vi "TrapezoidalMotionProfile.vi"(5 "MaxAccel":dbl=75.0, 7 "MaxVelocity":dbl=100.0, 8 "dt":u32=20, 9 "FinalVelocity":dbl, 10 "InitialVelocity":dbl, 11 "Distance":dbl=200.0) -> (0 "dt":u32=20, 1 "Accel":dbl[](array[numeric])=[0.0, 1.5, 3.0, 4.5, 6.0, 7.5, 9.0, 10.500000000000002, 12.0, 13.5, 15.0, 16.5, 18.0, 19.5, 21.000000000000004, 22.5, 24.0, 25.500000000000004, 27.0, 28.5, 30.0, 31.5, 33.0, 34.5, 36.0, 37.5, 39.0, 40.5, 42.00000000000001, 43.5, 45.0, 46.5, 48.0, 49.5, 51.00000000000001, 52.50000000000001, 54.0, 55.5, 57.0, 58.5, 60.0, 61.50000000000001, 63.0, 64.5, 66.0, 67.5, 69.0, 70.5, 72.0, 73.5, 75.0, 76.5, 78.0, 79.5, 81.0, 82.5, 84.00000000000001, 85.50000000000001, 87.0, 88.5, 90.0, 91.5, 93.0, 94.5, 96.0, 97.5, 99.0, 100.0, 100.0, 100.0, 100.0, 100.0, 100.0, 100.0, 100.0, 100.0, 100.0, 100.0, 100.0, 100.0, 100.0, 100.0, 100.0, 100.0, 100.0, 100.0, 100.0, 100.0, 100.0, 100.0, 100.0, 100.0, 100.0, 100.0, 100.0, 100.0, 100.0, 100.0, 100.0, 100.0, 100.0, 98.5, 97.0, 95.5, 94.0, 92.5, 91.0, 89.49999999999999, 87.99999999999999, 86.49999999999999, 84.99999999999999, 83.49999999999999, 81.99999999999999, 80.49999999999999, 78.99999999999999, 77.49999999999997, 76.00000000000001, 74.50000000000001, 73.00000000000001, 71.5, 70.0, 68.5, 67.0, 65.5, 64.0, 62.5, 61.0, 59.5, 57.99999999999999, 56.49999999999999, 54.99999999999999, 53.49999999999999, 51.99999999999999, 50.499999999999986, 48.999999999999986, 47.499999999999986, 45.999999999999986, 44.499999999999986, 42.999999999999986, 41.49999999999998, 39.99999999999998, 38.500000000000014, 37.000000000000014, 35.500000000000014, 34.000000000000014, 32.5, 31.0, 29.5, 28.0, 26.5, 25.0, 23.5, 22.0, 20.5, 19.0, 17.5, 15.999999999999986, 14.499999999999986, 12.999999999999986, 11.499999999999986, 9.999999999999986, 8.499999999999986, 6.999999999999986, 5.499999999999986, 3.999999999999986, 2.499999999999986, 0.9999999999999716, -0.4999999999999858], 2 "Vel":dbl[](array[numeric])=[0.0, 1.5, 3.0, 4.5, 6.0, 7.5, 9.0, 10.500000000000002, 12.0, 13.5, 15.0, 16.5, 18.0, 19.5, 21.000000000000004, 22.5, 24.0, 25.500000000000004, 27.0, 28.5, 30.0, 31.5, 33.0, 34.5, 36.0, 37.5, 39.0, 40.5, 42.00000000000001, 43.5, 45.0, 46.5, 48.0, 49.5, 51.00000000000001, 52.50000000000001, 54.0, 55.5, 57.0, 58.5, 60.0, 61.50000000000001, 63.0, 64.5, 66.0, 67.5, 69.0, 70.5, 72.0, 73.5, 75.0, 76.5, 78.0, 79.5, 81.0, 82.5, 84.00000000000001, 85.50000000000001, 87.0, 88.5, 90.0, 91.5, 93.0, 94.5, 96.0, 97.5, 99.0, 100.0, 100.0, 100.0, 100.0, 100.0, 100.0, 100.0, 100.0, 100.0, 100.0, 100.0, 100.0, 100.0, 100.0, 100.0, 100.0, 100.0, 100.0, 100.0, 100.0, 100.0, 100.0, 100.0, 100.0, 100.0, 100.0, 100.0, 100.0, 100.0, 100.0, 100.0, 100.0, 100.0, 100.0, 98.5, 97.0, 95.5, 94.0, 92.5, 91.0, 89.49999999999999, 87.99999999999999, 86.49999999999999, 84.99999999999999, 83.49999999999999, 81.99999999999999, 80.49999999999999, 78.99999999999999, 77.49999999999997, 76.00000000000001, 74.50000000000001, 73.00000000000001, 71.5, 70.0, 68.5, 67.0, 65.5, 64.0, 62.5, 61.0, 59.5, 57.99999999999999, 56.49999999999999, 54.99999999999999, 53.49999999999999, 51.99999999999999, 50.499999999999986, 48.999999999999986, 47.499999999999986, 45.999999999999986, 44.499999999999986, 42.999999999999986, 41.49999999999998, 39.99999999999998, 38.500000000000014, 37.000000000000014, 35.500000000000014, 34.000000000000014, 32.5, 31.0, 29.5, 28.0, 26.5, 25.0, 23.5, 22.0, 20.5, 19.0, 17.5, 15.999999999999986, 14.499999999999986, 12.999999999999986, 11.499999999999986, 9.999999999999986, 8.499999999999986, 6.999999999999986, 5.499999999999986, 3.999999999999986, 2.499999999999986, 0.9999999999999716, -0.4999999999999858], 3 "Pos":dbl[](array[numeric])=[0.0, 0.015000000000000001, 0.060000000000000005, 0.135, 0.24000000000000002, 0.37500000000000006, 0.54, 0.7350000000000001, 0.9600000000000001, 1.2149999999999999, 1.5000000000000002, 1.815, 2.16, 2.535, 2.9400000000000004, 3.375, 3.8400000000000003, 4.335000000000001, 4.859999999999999, 5.415, 6.000000000000001, 6.614999999999999, 7.26, 7.9350000000000005, 8.64, 9.375, 10.14, 10.935, 11.760000000000002, 12.614999999999998, 13.5, 14.415000000000001, 15.360000000000001, 16.335, 17.340000000000003, 18.375000000000004, 19.439999999999998, 20.535, 21.66, 22.815, 24.000000000000004, 25.215000000000003, 26.459999999999997, 27.734999999999996, 29.04, 30.375000000000004, 31.740000000000002, 33.135000000000005, 34.56, 36.015, 37.5, 39.015, 40.56, 42.135000000000005, 43.74, 45.37500000000001, 47.040000000000006, 48.735000000000014, 50.459999999999994, 52.214999999999996, 54.0, 55.815, 57.660000000000004, 59.535000000000004, 61.440000000000005, 63.37500000000001, 65.34, 67.33333333333334, 69.33333333333334, 71.33333333333334, 73.33333333333334, 75.33333333333333, 77.33333333333333, 79.33333333333333, 81.33333333333333, 83.33333333333333, 85.33333333333333, 87.33333333333334, 89.33333333333334, 91.33333333333334, 93.33333333333334, 95.33333333333334, 97.33333333333334, 99.33333333333334, 101.33333333333333, 103.33333333333333, 105.33333333333333, 107.33333333333333, 109.33333333333333, 111.33333333333334, 113.33333333333334, 115.33333333333334, 117.33333333333334, 119.33333333333334, 121.33333333333334, 123.33333333333334, 125.33333333333331, 127.33333333333333, 129.33333333333331, 131.33333333333331, 133.33333333333331, 135.31833333333338, 137.27333333333337, 139.19833333333338, 141.09333333333336, 142.95833333333337, 144.79333333333338, 146.59833333333336, 148.37333333333336, 150.11833333333337, 151.83333333333337, 153.51833333333337, 155.17333333333337, 156.79833333333337, 158.39333333333337, 159.95833333333337, 161.49333333333334, 162.99833333333333, 164.47333333333336, 165.91833333333335, 167.33333333333334, 168.71833333333336, 170.07333333333335, 171.39833333333334, 172.69333333333336, 173.95833333333334, 175.19333333333336, 176.39833333333337, 177.57333333333335, 178.71833333333336, 179.83333333333334, 180.91833333333335, 181.97333333333336, 182.99833333333336, 183.99333333333337, 184.95833333333334, 185.89333333333335, 186.79833333333335, 187.67333333333335, 188.51833333333335, 189.33333333333334, 190.11833333333334, 190.87333333333333, 191.59833333333333, 192.29333333333335, 192.95833333333334, 193.59333333333333, 194.19833333333335, 194.77333333333334, 195.31833333333333, 195.83333333333334, 196.31833333333333, 196.77333333333334, 197.19833333333335, 197.59333333333333, 197.95833333333334, 198.29333333333335, 198.59833333333333, 198.87333333333333, 199.11833333333334, 199.33333333333334, 199.51833333333335, 199.67333333333335, 199.79833333333335, 199.89333333333335, 199.95833333333334, 199.99333333333334, 199.99833333333333])   [LabVIEW 2016]
panel:
  out "Graph":dbl[][](graph)=[[0.0, 0.015000000000000001, 0.060000000000000005, 0.135, 0.24000000000000002, 0.37500000000000006, 0.54, 0.7350000000000001, 0.9600000000000001, 1.2149999999999999, 1.5000000000000002, 1.815, 2.16, 2.535, 2.9400000000000004, 3.375, 3.8400000000000003, 4.335000000000001, 4.859999999999999, 5.415, 6.000000000000001, 6.614999999999999, 7.26, 7.9350000000000005, 8.64, 9.375, 10.14, 10.935, 11.760000000000002, 12.614999999999998, 13.5, 14.415000000000001, 15.360000000000001, 16.335, 17.340000000000003, 18.375000000000004, 19.439999999999998, 20.535, 21.66, 22.815, 24.000000000000004, 25.215000000000003, 26.459999999999997, 27.734999999999996, 29.04, 30.375000000000004, 31.740000000000002, 33.135000000000005, 34.56, 36.015, 37.5, 39.015, 40.56, 42.135000000000005, 43.74, 45.37500000000001, 47.040000000000006, 48.735000000000014, 50.459999999999994, 52.214999999999996, 54.0, 55.815, 57.660000000000004, 59.535000000000004, 61.440000000000005, 63.37500000000001, 65.34, 67.33333333333334, 69.33333333333334, 71.33333333333334, 73.33333333333334, 75.33333333333333, 77.33333333333333, 79.33333333333333, 81.33333333333333, 83.33333333333333, 85.33333333333333, 87.33333333333334, 89.33333333333334, 91.33333333333334, 93.33333333333334, 95.33333333333334, 97.33333333333334, 99.33333333333334, 101.33333333333333, 103.33333333333333, 105.33333333333333, 107.33333333333333, 109.33333333333333, 111.33333333333334, 113.33333333333334, 115.33333333333334, 117.33333333333334, 119.33333333333334, 121.33333333333334, 123.33333333333334, 125.33333333333331, 127.33333333333333, 129.33333333333331, 131.33333333333331, 133.33333333333331, 135.31833333333338, 137.27333333333337, 139.19833333333338, 141.09333333333336, 142.95833333333337, 144.79333333333338, 146.59833333333336, 148.37333333333336, 150.11833333333337, 151.83333333333337, 153.51833333333337, 155.17333333333337, 156.79833333333337, 158.39333333333337, 159.95833333333337, 161.49333333333334, 162.99833333333333, 164.47333333333336, 165.91833333333335, 167.33333333333334, 168.71833333333336, 170.07333333333335, 171.39833333333334, 172.69333333333336, 173.95833333333334, 175.19333333333336, 176.39833333333337, 177.57333333333335, 178.71833333333336, 179.83333333333334, 180.91833333333335, 181.97333333333336, 182.99833333333336, 183.99333333333337, 184.95833333333334, 185.89333333333335, 186.79833333333335, 187.67333333333335, 188.51833333333335, 189.33333333333334, 190.11833333333334, 190.87333333333333, 191.59833333333333, 192.29333333333335, 192.95833333333334, 193.59333333333333, 194.19833333333335, 194.77333333333334, 195.31833333333333, 195.83333333333334, 196.31833333333333, 196.77333333333334, 197.19833333333335, 197.59333333333333, 197.95833333333334, 198.29333333333335, 198.59833333333333, 198.87333333333333, 199.11833333333334, 199.33333333333334, 199.51833333333335, 199.67333333333335, 199.79833333333335, 199.89333333333335, 199.95833333333334, 199.99333333333334, 199.99833333333333], [0.0, 1.5, 3.0, 4.5, 6.0, 7.5, 9.0, 10.500000000000002, 12.0, 13.5, 15.0, 16.5, 18.0, 19.5, 21.000000000000004, 22.5, 24.0, 25.500000000000004, 27.0, 28.5, 30.0, 31.5, 33.0, 34.5, 36.0, 37.5, 39.0, 40.5, 42.00000000000001, 43.5, 45.0, 46.5, 48.0, 49.5, 51.00000000000001, 52.50000000000001, 54.0, 55.5, 57.0, 58.5, 60.0, 61.50000000000001, 63.0, 64.5, 66.0, 67.5, 69.0, 70.5, 72.0, 73.5, 75.0, 76.5, 78.0, 79.5, 81.0, 82.5, 84.00000000000001, 85.50000000000001, 87.0, 88.5, 90.0, 91.5, 93.0, 94.5, 96.0, 97.5, 99.0, 100.0, 100.0, 100.0, 100.0, 100.0, 100.0, 100.0, 100.0, 100.0, 100.0, 100.0, 100.0, 100.0, 100.0, 100.0, 100.0, 100.0, 100.0, 100.0, 100.0, 100.0, 100.0, 100.0, 100.0, 100.0, 100.0, 100.0, 100.0, 100.0, 100.0, 100.0, 100.0, 100.0, 100.0, 98.5, 97.0, 95.5, 94.0, 92.5, 91.0, 89.49999999999999, 87.99999999999999, 86.49999999999999, 84.99999999999999, 83.49999999999999, 81.99999999999999, 80.49999999999999, 78.99999999999999, 77.49999999999997, 76.00000000000001, 74.50000000000001, 73.00000000000001, 71.5, 70.0, 68.5, 67.0, 65.5, 64.0, 62.5, 61.0, 59.5, 57.99999999999999, 56.49999999999999, 54.99999999999999, 53.49999999999999, 51.99999999999999, 50.499999999999986, 48.999999999999986, 47.499999999999986, 45.999999999999986, 44.499999999999986, 42.999999999999986, 41.49999999999998, 39.99999999999998, 38.500000000000014, 37.000000000000014, 35.500000000000014, 34.000000000000014, 32.5, 31.0, 29.5, 28.0, 26.5, 25.0, 23.5, 22.0, 20.5, 19.0, 17.5, 15.999999999999986, 14.499999999999986, 12.999999999999986, 11.499999999999986, 9.999999999999986, 8.499999999999986, 6.999999999999986, 5.499999999999986, 3.999999999999986, 2.499999999999986, 0.9999999999999716, -0.4999999999999858]]
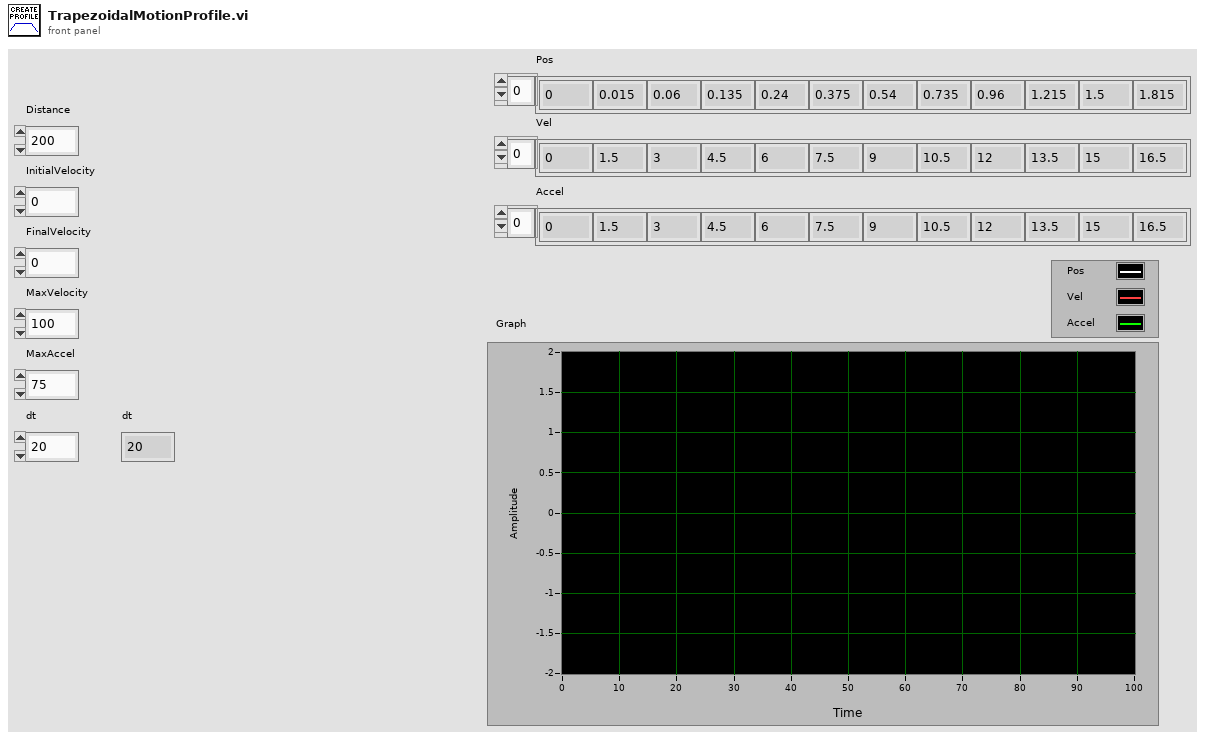
[diagram p1: front panel]
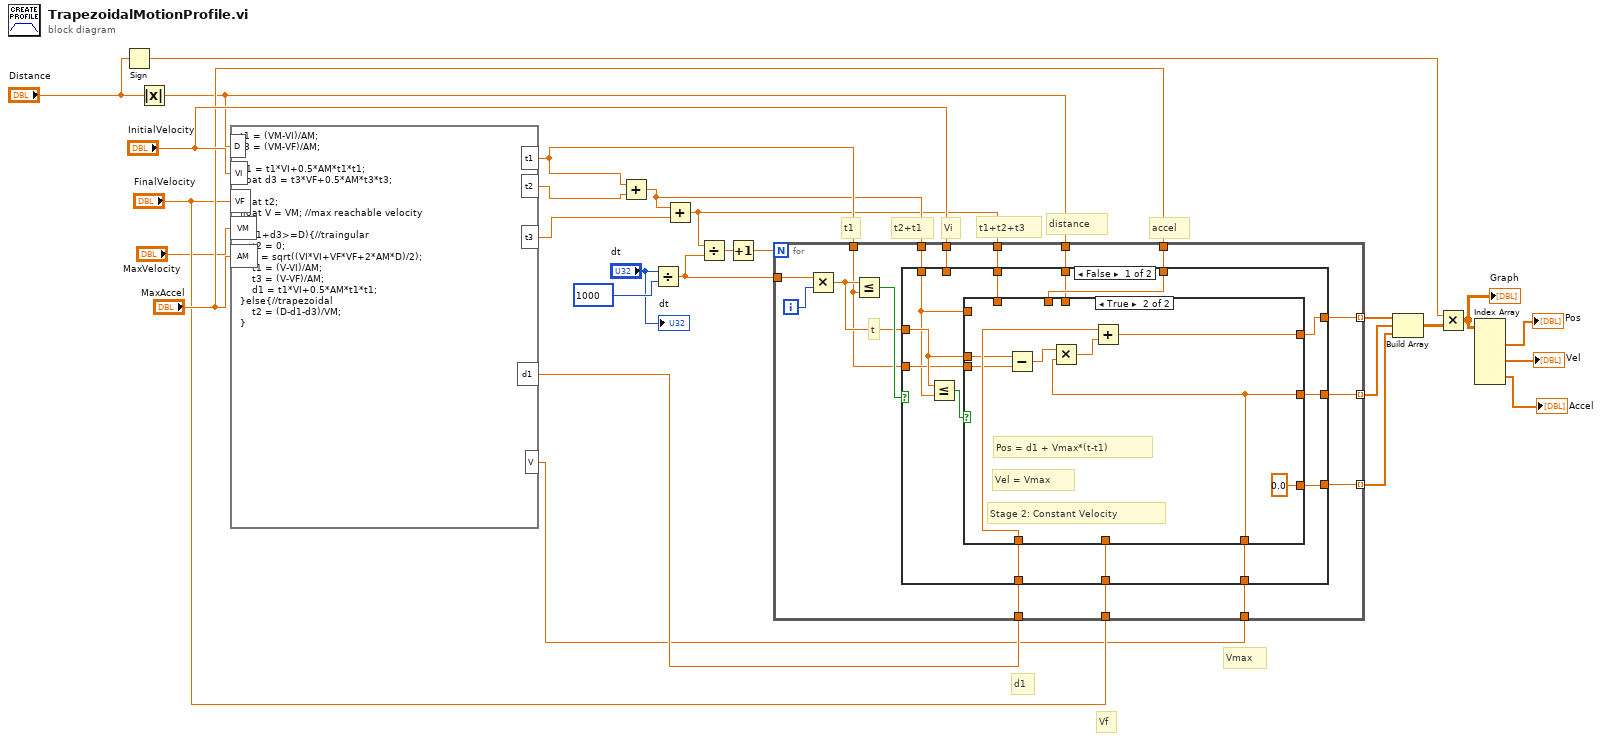
[diagram p0: block diagram]
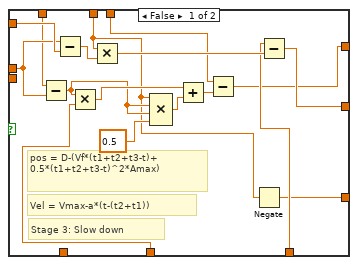
[diagram p2: hidden frame]
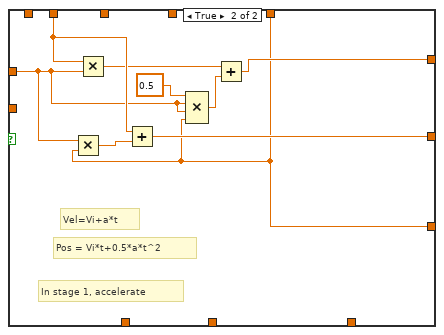
[diagram p3: hidden frame]
diagram:
  # "distance"
  # "Vf"
  # "t1+t2+t3"
  # "d1"
  # "Vmax"
  # "t1"
  # "t2+t1"
  # "Vi"
  # "accel"
  n1 = Sign(1:"Distance") -> (0:w5:dbl)
  n2 = Absolute Value(x="Distance") -> (abs(x)=w8:dbl)
  n3 = formula code="t1 = (VM-VI)/AM;\nt3 = (VM-VF)/AM;\n\nd1 = t1*VI+0.5*AM*t1*t1;\nfloat d3 = t3*VF+0.5*AM*t3*t3;\n\nfloat t2;\nfloat V = VM; //max reachable velocity\n\nif(d1+d3>=D){//traingular\n    t2 = 0;\n    V = sqrt((VI*VI+VF*VF+2*AM*D)/2);\n    t1 = (V-VI)/AM;\n    t3 = (V-VF)/AM;\n    d1 = t1*VI+0.5*AM*t1*t1;\n}else{//trapezoidal\n    t2 = (D-d1-d3)/VM;\n}"("VI"="InitialVelocity", "VF"="FinalVelocity", "D"=w8, "VM"="MaxVelocity", "AM"="MaxAccel") -> ("t1"=w21:dbl, "t3"=w26:dbl, "d1"=w17:dbl, "t2"=w27:dbl, "V"=w10:dbl)
  n4 = Add(x=w21, y=w27) -> (x+y=w18:dbl)
  n5 = Divide(x="dt", y=u32 1000) -> (x/y=w22:dbl)
  n6 = Add(x=w18, y=w26) -> (x+y=w14:dbl)
  n7 = Divide(x=w14, y=w22) -> (x/y=w24:dbl)
  n8 = Increment(x=w24) -> (x+1=w23:dbl)
  n9 = for {
    N: w23 -> [_]
    tunnel: w22 -> [w42]
    tunnel: w21 -> [w32]
    tunnel: "InitialVelocity" -> [w40]
    tunnel: "MaxAccel" -> [w39]
    tunnel: [w38] -> w15 mode=indexing
    tunnel: [w37] -> w16 mode=indexing
    tunnel: w18 -> [w36]
    tunnel: w10 -> [w34]
    tunnel: w17 -> [w33]
    tunnel: w14 -> [w31]
    tunnel: "FinalVelocity" -> [w30]
    tunnel: w8 -> [w29]
    tunnel: [w28] -> w9 mode=indexing
    i -> [w43]
    # "t"
    n10 = Multiply(x=w42, y=w43) -> (x*y=w35:dbl)
    n11 = Less Or Equal?(x=w35, y=w32) -> (x <= y?=w41:bool)
    n12 = case shown="False" w41 {
      tunnel: w40 -> [_ w88]
      tunnel: w39 -> [w48 w82]
      tunnel: w35 -> [w52 w85]
      tunnel: [w55 w89] -> w38
      tunnel: [w50 w83] -> w37
      tunnel: w36 -> [w49 _]
      tunnel: w34 -> [w54 _]
      tunnel: w33 -> [w53 _]
      tunnel: w32 -> [w51 _]
      tunnel: w31 -> [w47 _]
      tunnel: w30 -> [w46 _]
      tunnel: w29 -> [w45 _]
      tunnel: [w44 w82] -> w28
      frame False {
        n13 = Less Or Equal?(x=w52, y=w49) -> (x <= y?=w56:bool)
        n14 = case shown="True" w56 {
          tunnel: [w69 w78] -> w55
          tunnel: w54 -> [w70 w78]
          tunnel: w53 -> [_ w81]
          tunnel: w52 -> [w68 w80]
          tunnel: w51 -> [_ w79]
          tunnel: [w59 w75] -> w50
          tunnel: w49 -> [w73 _]
          tunnel: w48 -> [w57 _]
          tunnel: w47 -> [w67 _]
          tunnel: w46 -> [w66 _]
          tunnel: w45 -> [w60 _]
          tunnel: [w58 0.0] -> w44
          frame False {
            # "pos = D-(Vf*(t1+t2+t3-t)+\n0.5*(t1+t2+t3-t)^2*Amax)"
            # "Vel = Vmax-a*(t-(t2+t1))"
            # "Stage 3: Slow down"
            n15 = Subtract(x=w67, y=w68) -> (x-y=w63:dbl)
            n16 = Subtract(x=w68, y=w73) -> (x-y=w72:dbl)
            n17 = Multiply(x=w63, y=w66) -> (x*y=w65:dbl)
            n18 = Multiply(x=w57, y=w72) -> (x*y=w71:dbl)
            n19 = Compound Arithmetic op=MULTIPLY(w57, w63, w63, 0.5 ("value")) -> (w62:dbl)
            n20 = Add(x=w65, y=w62) -> (x+y=w61:dbl)
            n21 = Subtract(x=w60, y=w61) -> (x-y=w59:dbl)
            n22 = Negate(x=w57) -> (-x=w58:dbl)
            n23 = Subtract(x=w70, y=w71) -> (x-y=w69:dbl)
          }
          frame True {
            # "Pos = d1 + Vmax*(t-t1)"
            # "Vel = Vmax"
            # "Stage 2: Constant Velocity"
            n24 = Subtract(x=w80, y=w79) -> (x-y=w77:dbl)
            n25 = Multiply(x=w77, y=w78) -> (x*y=w76:dbl)
            n26 = Add(x=w81, y=w76) -> (x+y=w75:dbl)
          }
        }
      }
      frame True {
        # "Vel=Vi+a*t"
        # "Pos = Vi*t+0.5*a*t^2"
        # "In stage 1, accelerate"
        n27 = Multiply(x=w85, y=w82) -> (x*y=w90:dbl)
        n28 = Multiply(x=w88, y=w85) -> (x*y=w87:dbl)
        n29 = Add(x=w88, y=w90) -> (x+y=w89:dbl)
        n30 = Compound Arithmetic op=MULTIPLY(0.5 ("t2"), w85, w85, w82) -> (w84:dbl)
        n31 = Add(x=w87, y=w84) -> (x+y=w83:dbl)
      }
    }
  }
  n32 = Build Array(w16, w15, w9) -> (w6:dbl[][])
  n33 = Multiply(x=w5, y=w6) -> (x*y=w4:dbl[][])
  "Graph" <- w4
  n34 = Index Array(array=w4) -> (element #1=→"Pos":dbl[], element #2=→"Vel":dbl[], element #3=→"Accel":dbl[])  [unwired: 6 in]
  "dt" <- "dt"
